vi "read_tiff.vi"() -> ()   [LabVIEW 2014]
panel:
  out "Q_tags":u16
  out "is tiff big endian?":bool
  in  "Image_info":T1={"micro-position-xyz"={"micro-position_X_mm"=1.0, "micro-position Y_mm"=1.0, "micro-position Z_mm"=1.0}, "nano-position-xyz"={"nano-position_X_V"=1.0, "nano-position_Y_V"=1.0, "nano-position Z_V"=1.0}, "Kxyz"={"Kx_V/um"=1.0, "Ky_V/um"=1.0, "Kz_V/um"=1.0}, "image_size_x_um"=1.0, "image_size_y_um"=1.0, "Pixel_dwell_time_ms"=1.0, "Laser_power_V"=1.0, "Objective"="", "timestamp"=timestamp(0 s since 1904-01-01), "ColorMarkers"=[]}
  in  "image_array":sgl[][](array[numeric])
  in  "path_filename":path
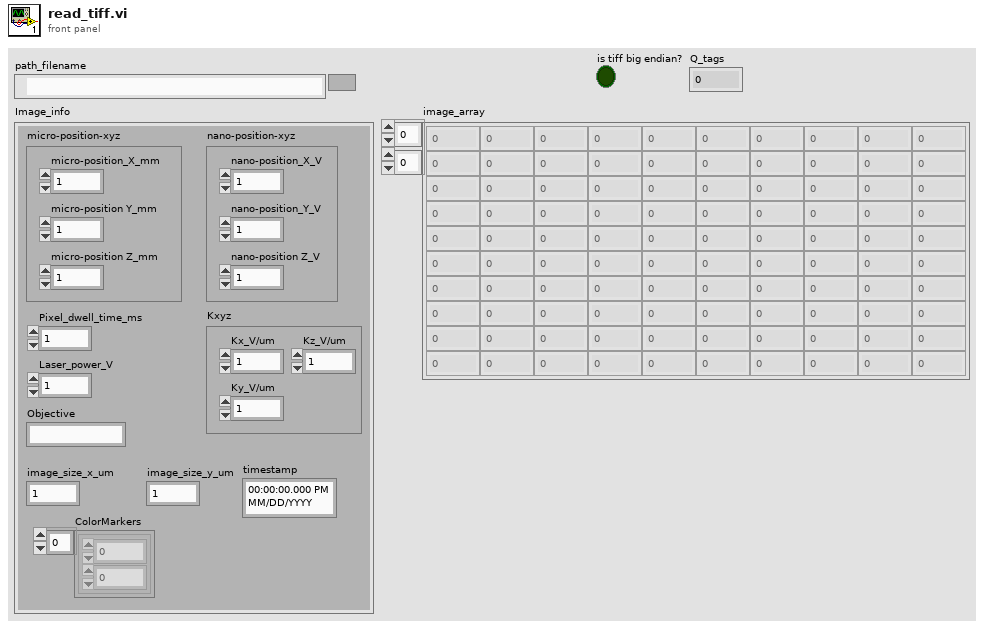
[diagram p1: front panel]
types:
  T1 = cluster{"micro-position-xyz":cluster{"micro-position_X_mm":sgl, "micro-position Y_mm":sgl, "micro-position Z_mm":sgl}, "nano-position-xyz":cluster{"nano-position_X_V":sgl, "nano-position_Y_V":sgl, "nano-position Z_V":sgl}, "Kxyz":cluster{"Kx_V/um":sgl, "Ky_V/um":sgl, "Kz_V/um":sgl}, "image_size_x_um":sgl, "image_size_y_um":sgl, "Pixel_dwell_time_ms":sgl, "Laser_power_V":sgl, "Objective":string, "timestamp":timestamp, "ColorMarkers":cluster{dbl, u32}[]}
  T2 = enum16{"open", "replace", "create", "open or create", "replace or create", "replace or create with confirmation"}
  T3 = enum16{"big-endian, network order", "native, host order", "little-endian"}
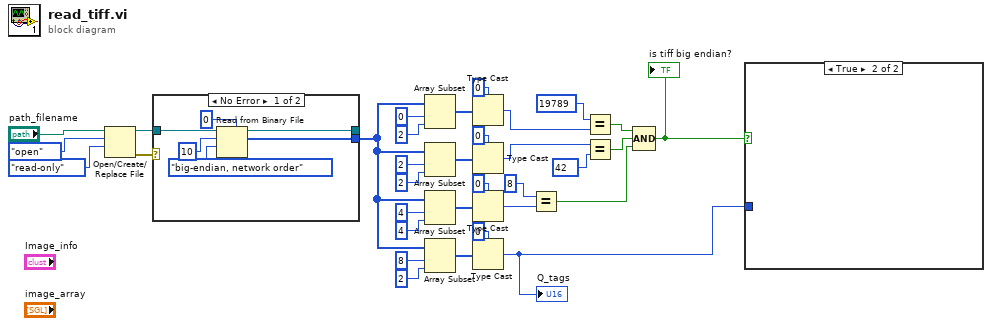
[diagram p0: block diagram]
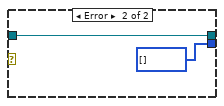
[diagram p3: hidden frame]
diagram:
  n1 = Open/Create/Replace File(file path (use dialog)="path_filename", operation (0:open)=T2."open", access (0:read/write)=enum16{"read/write", "read-only", "write-only"}."read-only") -> (refnum out=w29:refnum<file>, error out=w30:errorcluster)  [unwired: 3 in, 1 out]
  n2 = case shown="No Error" w30 {
    tunnel: w29 -> [w39 w41]
    tunnel: [w35 w41] -> _
    tunnel: [w34 u8[] []] -> w10
    frame No Error {
      n3 = Read from Binary File(5:u8 0 ("count (1)"), 9:T3."big-endian, network order" ("byte order (0:big-endian, network order)"), 10:10 ("count (1)"), 11:w39) -> (2:w34:u8[], 3:w35:refnum<file>)  [unwired: 2 in, 2 out]
    }
    frame Error {
    }
  }
  n4 = Array Subset(array=w10, index=0, length=2) -> (w18:u8[])
  n5 = Array Subset(array=w10, index=2, length=2) -> (w16:u8[])
  n6 = Array Subset(array=w10, index=4, length=4) -> (w25:u8[])
  n7 = Array Subset(array=w10, index=8, length=2) -> (w4:u8[])
  n8 = Type Cast(type=u16 0 ("index"), x=w18) -> (*(type *) &x=w15:u16)
  n9 = Type Cast(type=u16 0 ("index"), x=w16) -> (*(type *) &x=w14:u16)
  n10 = Type Cast(type=u32 0 ("index"), x=w25) -> (*(type *) &x=w9:u32)
  n11 = Type Cast(type=u16 0 ("index"), x=w4) -> (*(type *) &x=w1:u16)
  "Q_tags" <- w1
  n12 = Equal?(x=u32 8 ("index"), y=w9) -> (x = y?=w5:bool)
  n13 = Equal?(x=u16 19789, y=w15) -> (x = y?=w7:bool)
  n14 = Equal?(x=w14, y=u16 42 ("x")) -> (x = y?=w6:bool)
  n15 = Compound Arithmetic op=AND(w7, w6, w5) -> (w2:bool)
  "is tiff big endian?" <- w2
  n16 = case shown="True" w2 {
    tunnel: w1 -> [_ _]
    frame False {
    }
    frame True {
    }
  }
